vi "Write state.vi"(10 "state":T1(ring), 11 "Experiment in":refnum<class "Experiment.lvclass">) -> (3 "Experiment out":refnum<class "Experiment.lvclass">)   [LabVIEW 2013, in "Experiment.lvclass"]
uses:
  Experiment.lvclass
  Experiment.lvclass/Experiment.ctl
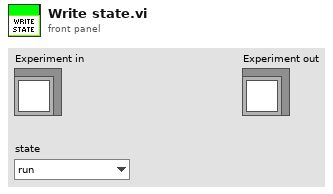
[diagram p1: front panel]
types:
  T1 = enum16{"run", "pause", "shutdown gracefully", "halt immediately"}
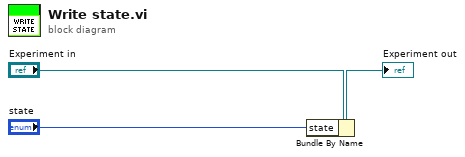
[diagram p0: block diagram]
diagram:
  n1 = Bundle By Name(cluster="Experiment in", "state"="state") -> (→"Experiment out":refnum<class "Experiment.lvclass">)
